vi "Check_String.vi"(5 "Surname":string, 6 "Action":T1(ring), 7 "Name":string, 8 "Error In":errorcluster, 9 "Instrument":string, 10 "Lab":string, 11 "Queue In":refnum<queue>) -> (0 "Error Out":errorcluster, 3 "Queue Out":refnum<queue>)   [LabVIEW 2021, in "Main.lvlib" / "Main_Programs_SubVIs.lvlib"]
doc: "This VI is used to check if the user did not entered information, if not message is queued to the QMH."
uses:
  Main_Programs_SubVIs.lvlib
  Tipski Definicii/Save_Sostojbi.ctl
  Polymorphic/Enq_Save_QMH.vi
  Polymorphic/Queues.lvlib
panel:
  # "Output"
  # "Input"
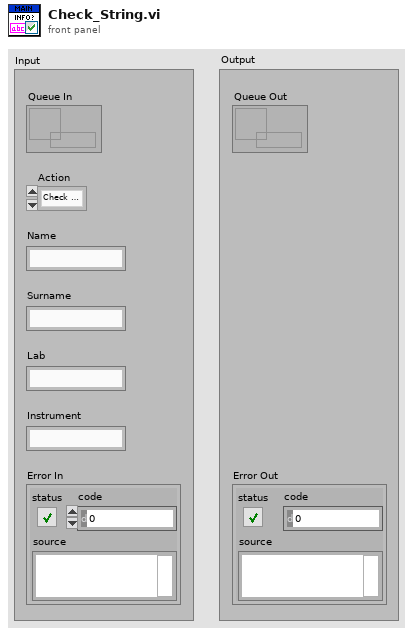
[diagram p1: front panel]
types:
  T1 = enum16{"Check Name", "Check Surname", "Check Lab", "Check Instrument"}
  T2 = typedef "Save_Sostojbi.ctl" = enum16{"Init", "Generate Message", "Pick Path", "Save", "End"}
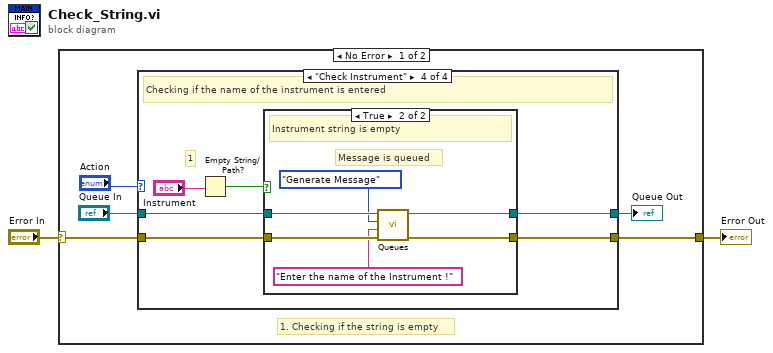
[diagram p0: block diagram]
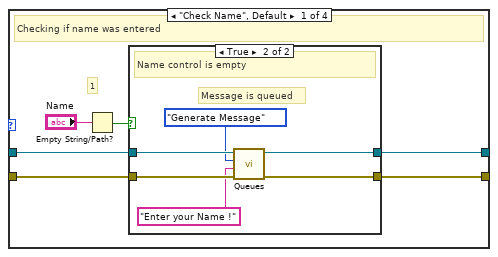
[diagram p2: hidden frame]
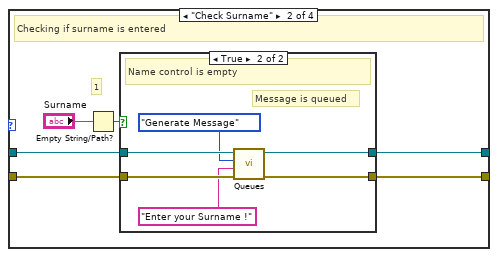
[diagram p4: hidden frame]
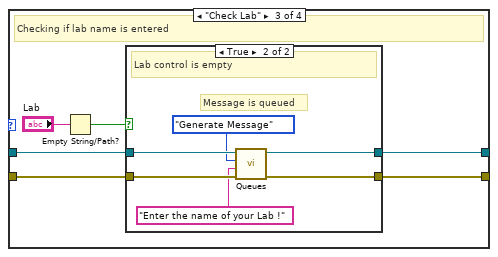
[diagram p6: hidden frame]
diagram:
  n1 = case shown="No Error" "Error In" {
    selector: "Error In" -> [w4 w64]
    tunnel: [w3 w64] -> w1
    frame No Error {
      # "1. Checking if the string is empty"
      n2 = case shown="\"Check Instrument\"" "Action" {
        tunnel: "Queue In" -> [w11 w24 w41 w53]
        tunnel: [w10 w27 w40 w52] -> w6
        tunnel: w4 -> [w9 w23 w37 w51]
        tunnel: [w8 w22 w36 w50] -> w3
        frame "Check Name", Default {
          # "1"
          # "Checking if name was entered"
          n3 = Empty String/Path?(string/path="Name") -> (empty?=w12:bool)
          n4 = case shown="True" w12 {
            tunnel: w11 -> [w15 w19]
            tunnel: [w15 w18] -> w10
            tunnel: w9 -> [w14 w21]
            tunnel: [w14 w20] -> w8
            frame False {
              # "Nothing happens"
              # "Name control is not empty"
            }
            frame True {
              # "Message is queued"
              # "Name control is empty"
              n5 = call-poly "Queues.vi"("Error In"=w21, "Message"="Enter your Name !", "Instruction"=Save_Sostojbi."Generate Message", "Queue In"=w19) -> ("Error Out"=w20:errorcluster, "Queue Out"=w18:refnum<queue>)  [unwired: 6 in]
            }
          }
        }
        frame "Check Surname" {
          # "1"
          # "Checking if surname is entered"
          n6 = Empty String/Path?(string/path="Surname") -> (empty?=w25:bool)
          n7 = case shown="True" w25 {
            tunnel: w24 -> [w29 w33]
            tunnel: [w29 w32] -> w27
            tunnel: w23 -> [w28 w35]
            tunnel: [w28 w34] -> w22
            frame False {
              # "Nothing happends"
              # "Name control is not empty"
            }
            frame True {
              # "Message is queued"
              # "Name control is empty"
              n8 = call-poly "Queues.vi"("Error In"=w35, "Message"="Enter your Surname !", "Instruction"=Save_Sostojbi."Generate Message", "Queue In"=w33) -> ("Error Out"=w34:errorcluster, "Queue Out"=w32:refnum<queue>)  [unwired: 6 in]
            }
          }
        }
        frame "Check Lab" {
          # "Checking if lab name is entered"
          n9 = Empty String/Path?(string/path="Lab") -> (empty?=w38:bool)
          n10 = case shown="True" w38 {
            tunnel: w41 -> [w42 w47]
            tunnel: [w42 w46] -> w40
            tunnel: w37 -> [w43 w49]
            tunnel: [w43 w48] -> w36
            frame False {
              # "Nothing happends"
              # "Lab control is not empty"
            }
            frame True {
              # "Message is queued"
              # "Lab control is empty"
              n11 = call-poly "Queues.vi"("Error In"=w49, "Message"="Enter the name of your Lab !", "Instruction"=Save_Sostojbi."Generate Message", "Queue In"=w47) -> ("Error Out"=w48:errorcluster, "Queue Out"=w46:refnum<queue>)  [unwired: 6 in]
            }
          }
        }
        frame "Check Instrument" {
          # "1"
          # "Checking if the name of the instrument is entered"
          n12 = Empty String/Path?(string/path="Instrument") -> (empty?=w55:bool)
          n13 = case shown="True" w55 {
            tunnel: w53 -> [w57 w61]
            tunnel: [w57 w60] -> w52
            tunnel: w51 -> [w56 w63]
            tunnel: [w56 w62] -> w50
            frame False {
              # "Nothing happends"
              # "Instrument string is not empty"
            }
            frame True {
              # "Message is queued"
              # "Instrument string is empty"
              n14 = call-poly "Queues.vi"("Error In"=w63, "Message"="Enter the name of the Instrument !", "Instruction"=Save_Sostojbi."Generate Message", "Queue In"=w61) -> ("Error Out"=w62:errorcluster, "Queue Out"=w60:refnum<queue>)  [unwired: 6 in]
            }
          }
        }
      }
      "Queue Out" <- w6
    }
    frame Error {
    }
  }
  "Error Out" <- w1
